vi "Test_MergeErrorsPublication_ErrorArray_1stErrorMerged.vi"(8 "error in (no error)":errorcluster, 11 "TestCase in":refnum<class "TestPublicationPolicy.lvclass">) -> (0 "error out":errorcluster, 3 "TestCase out":refnum<class "TestPublicationPolicy.lvclass">)   [LabVIEW 2015, in "PublicationPolicy.lvlib" / "TestPublicationPolicy.lvclass"]
uses:
  TestPublicationPolicy.lvclass
  MergeErrorsPublication/MergeErrorsPublication.lvclass
  IMediator/IPublicationPolicy/IPublicationPolicy.lvclass
  Transport/QueueTransport/QueueTransport.lvclass/QueueTransport.ctl
  IMediator/PublishRequest/PublishRequest.lvclass/PublishRequest.ctl
  IMediator/MutexedPublishRequest/MutexedPublishRequest.lvclass/MutexedPublishRequest.ctl
  IMediator/PublishRequest/Write Publish Request Data.vi
  <vilib>/Utility/error.llb/Error Cluster From Error Code.vi
  Transport/QueueTransport/QueueTransport.lvclass
  IMediator/MutexedPublishRequest/MutexedPublishRequest.lvclass
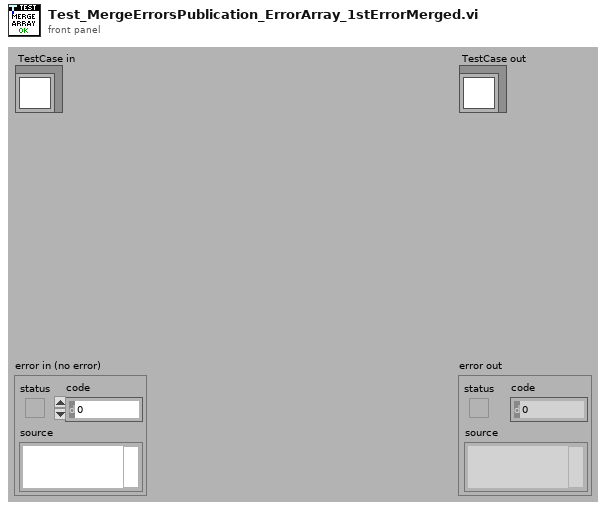
[diagram p1: front panel]
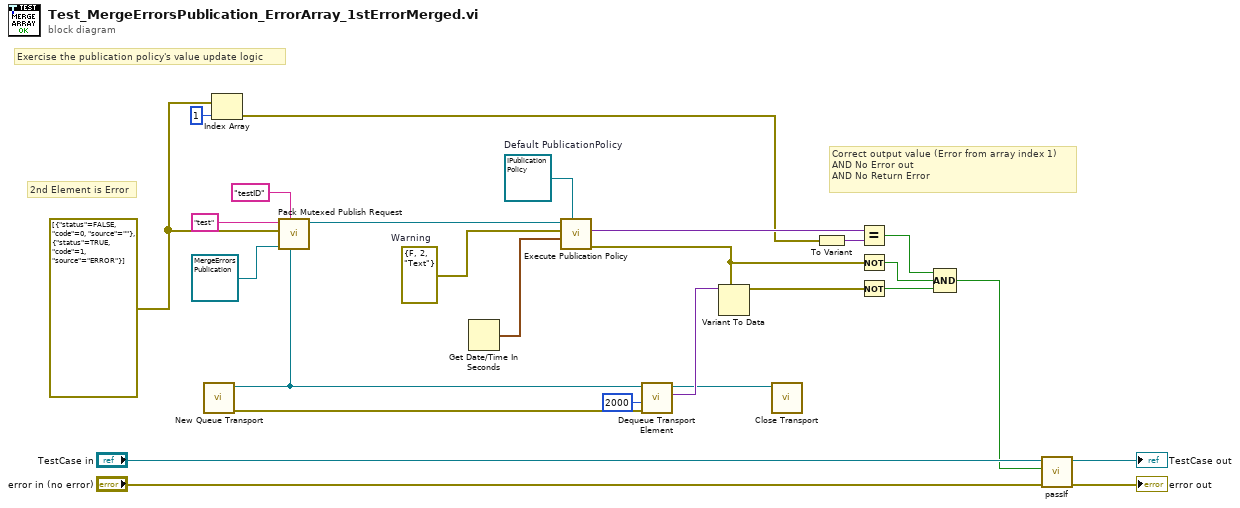
[diagram p0: block diagram]
diagram:
  w3 = errorcluster[] [{"status"=FALSE, "code"=0, "source"=""}, {"status"=TRUE, "code"=1, "source"="ERROR"}] ("error constant")
  w20 = refnum<class "IPublicationPolicy.lvclass"> refnum  # Default PublicationPolicy
  w4 = errorcluster {"status"=FALSE, "code"=2, "source"="Text"}  # Warning
  # "2nd Element is Error"
  # "Correct output value (Error from array index 1)\nAND No Error out\nAND No Return Error"
  # "Exercise the publication policy's value update logic"
  n1 = call "New Queue Transport.vi"() -> ("error out"=w16:errorcluster, "QueueTransport"=w17:refnum<class "QueueTransport.lvclass">)  [unwired: 10 in]
  n2 = Index Array(array=w3, index=1) -> (element=w1:errorcluster)
  n3 = call "Pack Mutexed Publish Request.vi"("Return Error Transport"=w17, "Publisher ID"="testID", "PublicationPolicy"=refnum<class "MergeErrorsPublication.lvclass"> refnum ("PublicationPolicy.lvlib:MergeErrorsPublication.lvclass"), "Datum Value or Type"=w3, "Datum Name"="test") -> ("MutexedPublishRequest Out"=w22:refnum<class "MutexedPublishRequest.lvclass">)  [unwired: 6 in]
  n4 = Get Date/Time In Seconds() -> (seconds since 1Jan1904=w23:timestamp)
  n5 = call-dynamic "Execute Publication Policy.vi"("Default PublicationPolicy"=w20, "Last Publish Time"=w23, "Last Published Value"=w4, "MutexedPublishRequest"=w22) -> ("error out (Reject Publication)"=w7:errorcluster, "Value to Publish"=w13:variant)  [unwired: 5 in, 1 out]
  n6 = call "Dequeue Transport Element.vi"("error in (no error)"=w16, "Timeout In ms (-1)"=2000, "QueueTransport in"=w17) -> ("Data"=w14:variant, "QueueTransport out"=w10:refnum<class "QueueTransport.lvclass">)  [unwired: 5 in, 2 out]
  n7 = Variant To Data(type=w7, Variant=w14) -> (data=w11:errorcluster)  [unwired: 1 in, 1 out]
  n8 = call-dynamic "Close Transport.vi"("QueueTransport in"=w10) -> ()  [unwired: 10 in, 1 out]
  n9 = To Variant(anything=w1) -> (Variant=w12:variant)
  n10 = Equal?(x=w13, y=w12) -> (x = y?=w9:bool)
  n11 = Not(x=w7) -> (.not. x?=w6:bool)
  n12 = Not(x=w11) -> (.not. x?=w8:bool)
  n13 = Compound Arithmetic op=AND(w9, w6, w8) -> (w5:bool)
  n14 = call-dynamic "passIf.vi"("error in (no error)"="error in (no error)", "pass"=w5, "TestCase in"="TestCase in") -> ("error out"=→"error out":errorcluster, "TestCase out"=→"TestCase out":refnum<class "TestPublicationPolicy.lvclass">)  [unwired: 7 in]
